vi "rapid_temp_control.vi"() -> ()   [LabVIEW 2009]
uses:
  <vilib>/Utility/error.llb/DialogType.ctl
  <vilib>/DAQmx/create/timing.llb/DAQmx Create Timing Source.vi
  <vilib>/DAQmx/create/timing.llb/DAQmx Create Timing Source (Control Loop From Task).vi
  <vilib>/DAQmx/read.llb/DAQmx Read (Analog 1D Wfm NChan NSamp).vi
  <vilib>/Platform/TimedLoop/XDataNode/XDataNode.xnode
  <vilib>/Platform/TimedLoop/XDataNode/loadlvalarms.vi
  <vilib>/Platform/TimedLoop/XDataNode/timing_clust.ctl
  <vilib>/Platform/TimedLoop/XDataNode/nitl_modes.ctl
  <vilib>/Platform/TimedLoop/XDataNode/wakeup.ctl
  Program Files/National Instruments/LabVIEW 2009/examples/DAQmx/Control/Control.llb/Proportional Gain.vi
  <vilib>/DAQmx/write.llb/DAQmx Write (Analog 1D DBL 1Chan NSamp).vi
  <vilib>/Platform/TimedLoop/XDataNode/XDNodeRunTimeDep.lvlib
panel:
  in  "exit":bool
  in  "waveform2play":dbl[](array[numeric]) format="%0.2f"
  in  "Run mode":enum16{"idle", "record", "play"}(ring)
  out "Measurement":waveform(dbl)[](graph)
  in  "Maximum Value":dbl=10.0 caption="AI Maximum Value" format="%0.2f"
  in  "Minimum Value":dbl=-10.0 caption="AI Minimum Value" format="%0.2f"
  in  "rate":dbl=1000.0 format="%0.2f"
  in  "Physical Channels":tag="Dev1/ao0:1"
  in  "stop":bool
  in  "Proportional Gain":dbl=1.0
  in  "Set Point":dbl
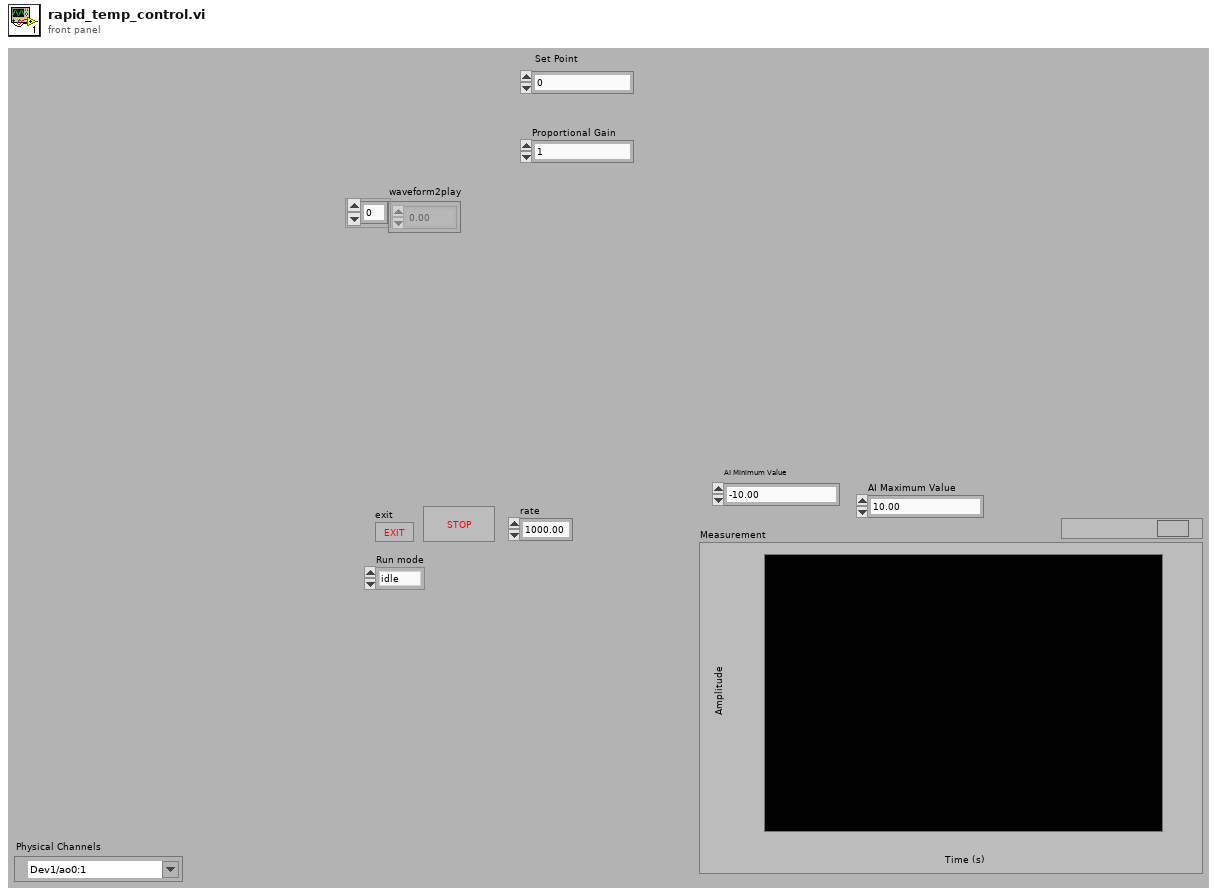
[diagram p1: front panel]
types:
  T1 = typedef "XDNodeRunTimeDep.lvlib/timing_clust.ctl" = cluster{"Expected End [f-1]":u64, "Actual End [f-1]":u64, "Finished Late? [f-1]":bool, "Expected End [i-1]":u64, "Actual End [i-1]":u64, "Finished Late? [i-1]":bool, "Expected Start [i]":u64, "Actual Start [i]":u64, "Expected Start [f]":u64, "Actual Start [f]":u64, "Source Name":string, "Structure Name":string, "Period":i64, "Deadline":i64, "Offset":i64, "Start":i64, "Priority":i32, "Timeout":i32, "Mode":T2, "Wakeup Reason":T3, "Error":errorcluster, "Source Type":string, "Secondary Source Type":string, "Global End Time":u64, "Global Start Time":u64, "Frame Duration":u64, "Iteration Duration":u64, "Assigned CPU":i32, "I/O Scan Engine Mode":u32}
  T2 = typedef "XDNodeRunTimeDep.lvlib/nitl_modes.ctl" = enum32{"No Change", "Process missed periods, maintain original phase", "Discard missed periods, maintain original phase", "Process missed periods, ignore original phase", "Discard missed periods, ignore original phase"}
  T3 = typedef "XDNodeRunTimeDep.lvlib/wakeup.ctl" = enum32{"Normal", "Aborted", "Asynchronous wakeup", "Timing source error", "Timed loop error", "Timeout"}
  T4 = typedef "DialogType.ctl" = u16
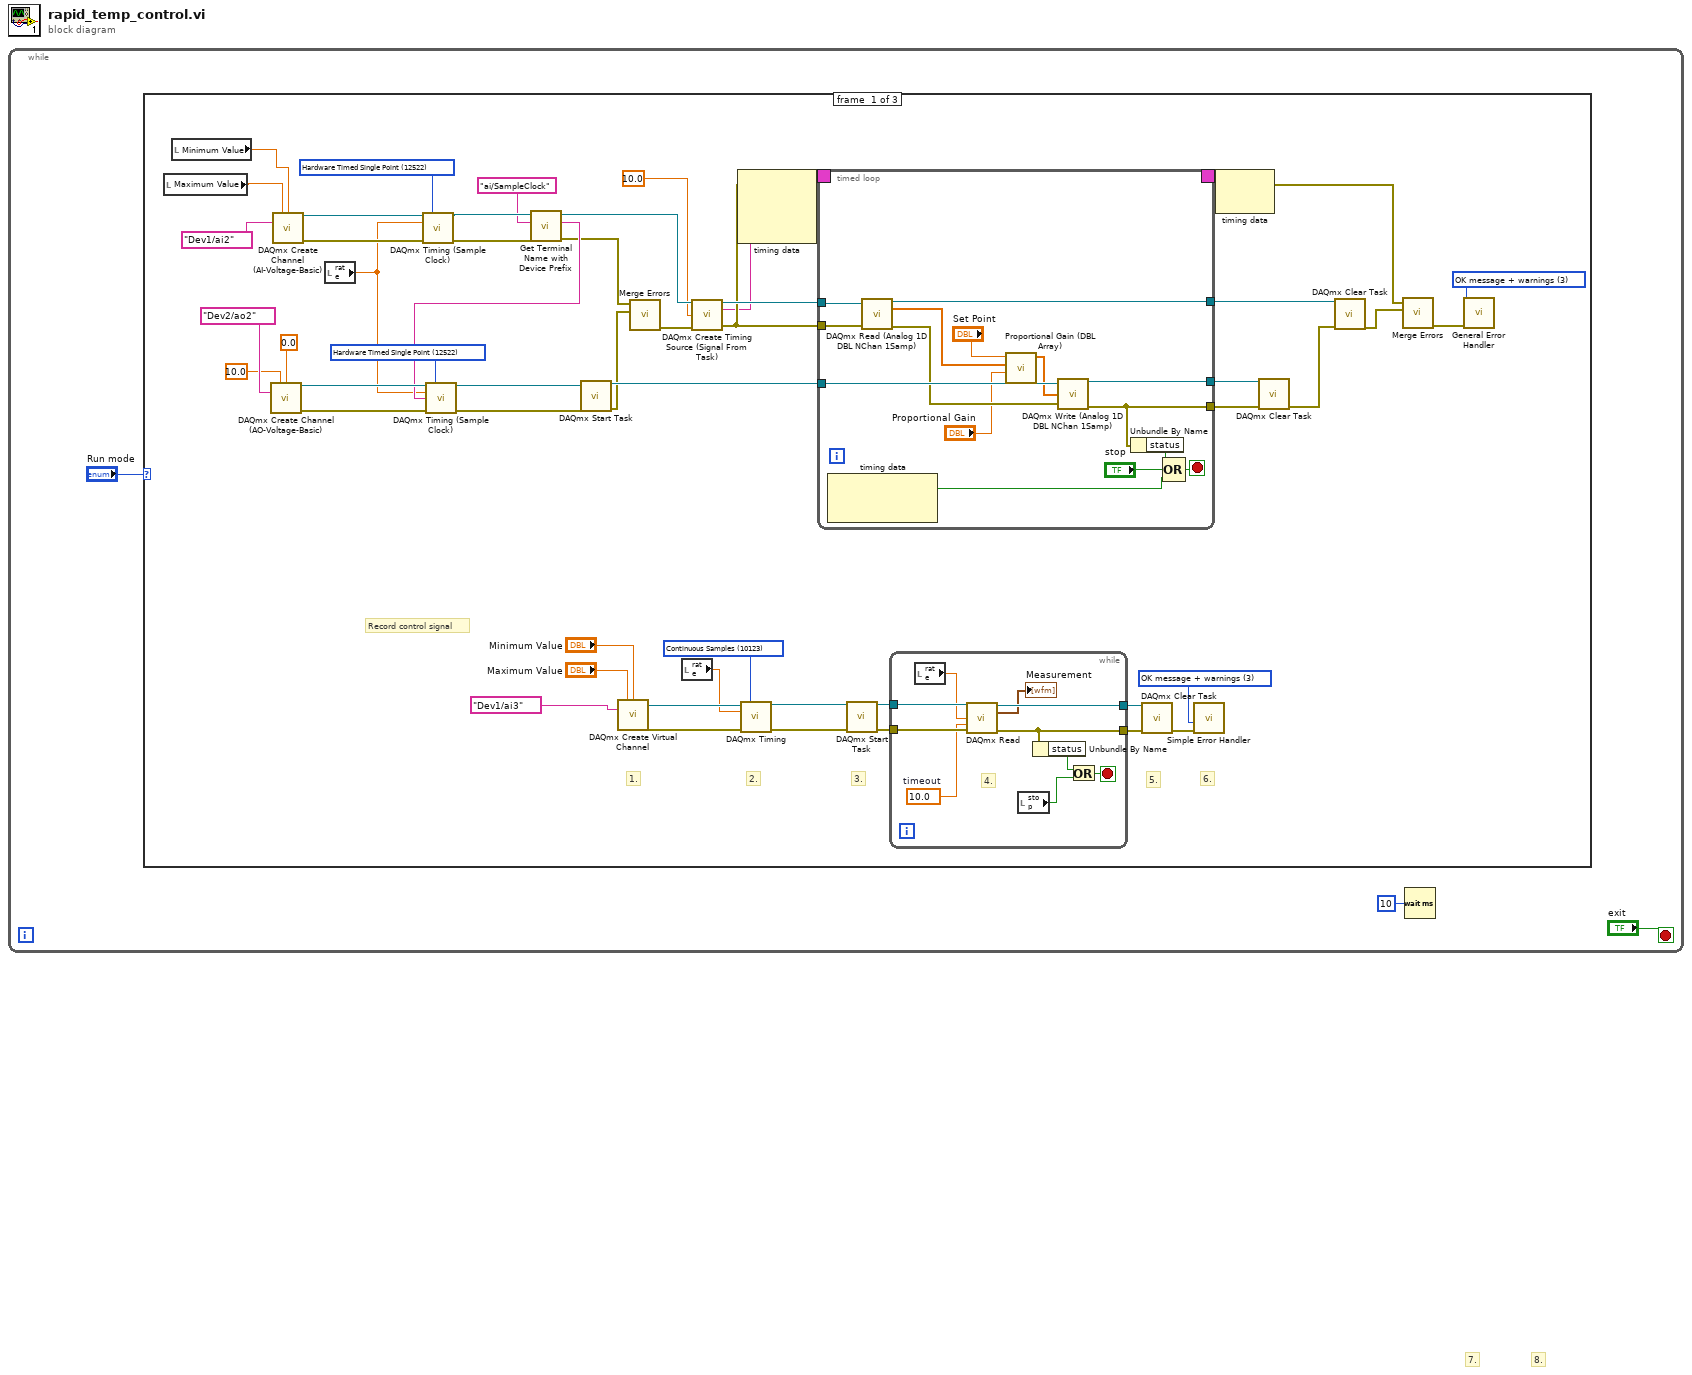
[diagram p0: block diagram]
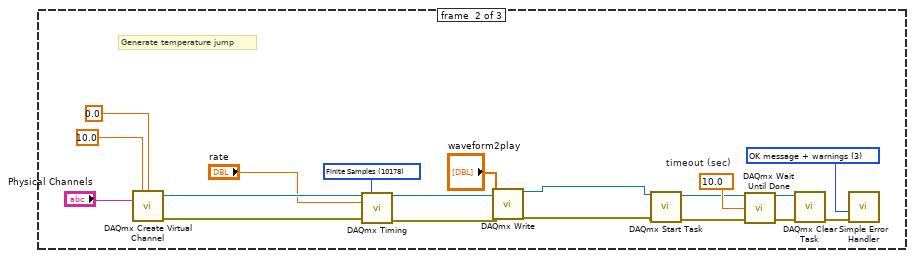
[diagram p2: hidden frame]
diagram:
  # "7."
  # "8."
  n1 = while {
    stop <- "exit" stop-if-true
    n2 = case shown="\"idle\", Default" "Run mode" {
      frame #0 {
        w8 = T4 3 items=["no dialog", "OK message", "continue or stop message", "OK message + warnings", "continue/stop + warnings"] ("type of dialog (OK msg:1)")
        w12 = 10123 items=["Finite Samples"=10178, "Continuous Samples"=10123] ("sample mode")
        w40 = 12522 items=["Finite Samples"=10178, "Continuous Samples"=10123, "Hardware Timed Single Point"=12522] ("sample mode")
        w41 = 12522 items=["Finite Samples"=10178, "Continuous Samples"=10123, "Hardware Timed Single Point"=12522] ("sample mode")
        w44 = T4 3 items=["no dialog", "OK message", "continue or stop message", "OK message + warnings", "continue/stop + warnings"] ("type of dialog (OK msg:1)")
        # "6."
        # "5."
        # "3."
        # "2."
        # "1."
        # "Record control signal"
        n3 = local read "Maximum Value"() -> (w5:dbl)
        n4 = local read "Minimum Value"() -> (w4:dbl)
        n5 = call-poly <vilib>:"DAQmx Create Channel (AO-Voltage-Basic).vi"("maximum value"=10.0 ("Maximum Value"), "minimum value"=0.0 ("Minimum Value"), "physical channels"=tag "Dev2/ao2" ("Physical Channels")) -> ("task out"=w48:refnum<k21>, "error out"=w47:errorcluster)  [unwired: 11 in]
        n6 = call-poly <vilib>:"DAQmx Create Channel (AI-Voltage-Basic).vi"("maximum value"=w5, "minimum value"=w4, "physical channels"=tag "Dev1/ai2" ("Physical Channels 2")) -> ("task out"=w52:refnum<k21>, "error out"=w53:errorcluster)  [unwired: 11 in]
        n7 = local read "rate"() -> (w6:dbl)
        n8 = call-poly <vilib>:"DAQmx Timing (Sample Clock).vi"("task/channels in"=w52, "sample mode"=w41, "rate"=w6, "error in"=w53) -> ("task out"=w30:refnum<k21>, "error out"=w27:errorcluster)  [unwired: 10 in]
        n9 = call "Get Terminal Name with Device Prefix.vi"("error in (no error)"=w27, "Local Terminal Name"="ai/SampleClock", "task/channels in"=w30) -> ("error out"=w26:errorcluster, "Terminal Name with Device Prefix"=w28:tag, "task out"=w29:refnum<k21>)  [unwired: 6 in]
        n10 = call-poly <vilib>:"DAQmx Timing (Sample Clock).vi"("task/channels in"=w48, "sample mode"=w40, "rate"=w6, "source"=w28, "error in"=w47) -> ("task out"=w25:refnum<k21>, "error out"=w24:errorcluster)  [unwired: 9 in]
        n11 = call <vilib>:"DAQmx Start Task.vi"("task/channels in"=w25, "error in"=w24) -> ("task out"=w46:refnum<k21>, "error out"=w42:errorcluster)  [unwired: 12 in]
        n12 = call-poly <vilib>:"DAQmx Create Virtual Channel.vi"("maximum value"="Maximum Value", "minimum value"="Minimum Value", "physical channels"=tag "Dev1/ai3" ("Physical Channel")) -> ("task out"=w16:refnum<k21>, "error out"=w19:errorcluster)  [unwired: 11 in]
        n13 = call <vilib>:"Merge Errors.vi"("error in 2 (no error)"=w42, "error in 1 (no error)"=w26) -> ("error out"=w39:errorcluster)  [unwired: 5 in]
        n14 = local read "rate"() -> (w7:dbl)
        n15 = call-poly "DAQmx Create Timing Source (Signal From Task).vi"("task/channels in"=w29, "sleep time (us)"=10.0, "error in"=w39) -> ("task out"=w38:refnum<k21>, "timing source out"=w32:string, "error out"=w33:errorcluster)  [unwired: 10 in]
        n16 = node-c288(w33, w32) -> (w56:T1)  [unwired: 1 in]
        n17 = call-poly <vilib>:"DAQmx Timing.vi"("task/channels in"=w16, "sample mode"=w12, "rate"=w7, "error in"=w19) -> ("task out"=w11:refnum<k21>, "error out"=w10:errorcluster)  [unwired: 10 in]
        n18 = timed-loop {
          timing-out: [_] -> w55
          timing: w56 -> [_]
          tunnel: [w72] -> w37
          tunnel: w33 -> [w77]
          tunnel: w38 -> [w78]
          tunnel: [w79] -> w45
          tunnel: w46 -> [w80]
          tunnel: [w81] -> w54
          stop <- w75 stop-if-true
          n19 = node-c288() -> (w71:bool)  [unwired: 1 in, 1 out]
          n20 = call-poly <vilib>:"DAQmx Read (Analog 1D DBL NChan 1Samp).vi"("task/channels in"=w78, "error in"=w77) -> ("task out"=w81:refnum<k21>, "data"=w69:dbl[], "error out"=w73:errorcluster)  [unwired: 11 in]
          n21 = call-poly "Proportional Gain (DBL Array).vi"("Proportional Gain"="Proportional Gain", "Process Variable"=w69, "Set Point"="Set Point") -> ("Output Value"=w70:dbl[])  [unwired: 8 in]
          n22 = call-poly <vilib>:"DAQmx Write (Analog 1D DBL NChan 1Samp).vi"("task/channels in"=w80, "data"=w70, "error in"=w73) -> ("task out"=w79:refnum<k21>, "error out"=w72:errorcluster)  [unwired: 10 in, 1 out]
          n23 = Unbundle By Name(w72) -> ("status"=w76:bool)
          n24 = Compound Arithmetic op=OR(w76, "stop", w71) -> (w75:bool)
        }
        n25 = call <vilib>:"DAQmx Start Task.vi"("task/channels in"=w11, "error in"=w10) -> ("task out"=w15:refnum<k21>, "error out"=w18:errorcluster)  [unwired: 12 in]
        n26 = while {
          tunnel: w18 -> [w66]
          tunnel: w15 -> [w65]
          tunnel: [w64] -> w14
          tunnel: [w62] -> w9
          stop <- w60 stop-if-true
          w59 = 10.0  # timeout
          # "4."
          n27 = local read "rate"() -> (w58:dbl)
          n28 = call-poly <vilib>:"DAQmx Read.vi"("task/channels in"=w65, "number of samples per channel"=w58, "timeout"=w59, "error in"=w66) -> ("task out"=w64:refnum<k21>, "data"=→"Measurement":waveform(dbl)[], "error out"=w62:errorcluster)  [unwired: 9 in]
          n29 = local read "stop"() -> (w57:bool)
          n30 = Unbundle By Name(w62) -> ("status"=w61:bool)
          n31 = Or(x=w61, y=w57) -> (x .or. y?=w60:bool)
        }
        n32 = call <vilib>:"DAQmx Clear Task.vi"("task in"=w14, "error in"=w9) -> ("error out"=w17:errorcluster)  [unwired: 13 in]
        n33 = call <vilib>:"Simple Error Handler.vi"("type of dialog (OK msg:1)"=w8, "error in (no error)"=w17) -> ()  [unwired: 3 in, 5 out]
        n34 = node-c288(w55) -> (w31:errorcluster)
        n35 = call <vilib>:"DAQmx Clear Task.vi"("task in"=w45, "error in"=w37) -> ("error out"=w36:errorcluster)  [unwired: 13 in]
        n36 = call <vilib>:"DAQmx Clear Task.vi"("task in"=w54, "error in"=w36) -> ("error out"=w35:errorcluster)  [unwired: 13 in]
        n37 = call <vilib>:"Merge Errors.vi"("error in 2 (no error)"=w35, "error in 1 (no error)"=w31) -> ("error out"=w34:errorcluster)  [unwired: 5 in]
        n38 = call <vilib>:"General Error Handler.vi"("type of dialog (OK msg:1)"=w44, "error in (no error)"=w34) -> ()  [unwired: 9 in, 5 out]
      }
      frame #1 {
        w104 = T4 3 items=["no dialog", "OK message", "continue or stop message", "OK message + warnings", "continue/stop + warnings"] ("type of dialog (OK msg:1)")
        w103 = 10.0  # timeout (sec)
        w92 = 10178 items=["Finite Samples"=10178, "Continuous Samples"=10123] ("sample mode")
        # "Generate temperature jump"
        n39 = call-poly <vilib>:"DAQmx Create Virtual Channel.vi"("maximum value"=10.0 ("Maximum Value"), "minimum value"=0.0 ("Minimum Value"), "physical channels"="Physical Channels") -> ("task out"=w108:refnum<k21>, "error out"=w109:errorcluster)  [unwired: 11 in]
        n40 = call-poly <vilib>:"DAQmx Timing.vi"("task/channels in"=w108, "sample mode"=w92, "rate"="rate", "error in"=w109) -> ("task out"=w96:refnum<k21>, "error out"=w97:errorcluster)  [unwired: 10 in]
        n41 = call-poly <vilib>:"DAQmx Write.vi"("task/channels in"=w96, "data"="waveform2play", "error in"=w97) -> ("task out"=w105:refnum<k21>, "error out"=w106:errorcluster)  [unwired: 10 in, 1 out]
        n42 = call <vilib>:"DAQmx Start Task.vi"("task/channels in"=w105, "error in"=w106) -> ("task out"=w98:refnum<k21>, "error out"=w99:errorcluster)  [unwired: 12 in]
        n43 = call <vilib>:"DAQmx Wait Until Done.vi"("task/channels in"=w98, "timeout (sec)"=w103, "error in"=w99) -> ("task out"=w102:refnum<k21>, "error out"=w101:errorcluster)  [unwired: 11 in]
        n44 = call <vilib>:"DAQmx Clear Task.vi"("task in"=w102, "error in"=w101) -> ("error out"=w100:errorcluster)  [unwired: 13 in]
        n45 = call <vilib>:"Simple Error Handler.vi"("type of dialog (OK msg:1)"=w104, "error in (no error)"=w100) -> ()  [unwired: 3 in, 5 out]
      }
      frame #2 {
      }
    }
    n46 = Wait (ms)(milliseconds to wait=u32 10) -> ()  [unwired: 1 out]
  }
